vi "Control_cmd.vi"(6 "Arty-7 Error In":errorcluster, 7 "Control Command":u8 format="%b", 8 "Arty-7 VISA In":refnum<visa-resource-name>) -> (0 "Arty-7 Error out":errorcluster, 2 "WrReg Status":string, 3 "WrReg Done":bool, 5 "Arty-7 VISA out":refnum<visa-resource-name>)   [LabVIEW 2019]
uses:
  <vilib>/Utility/error.llb/DialogType.ctl
  Board_Global_Var.vi
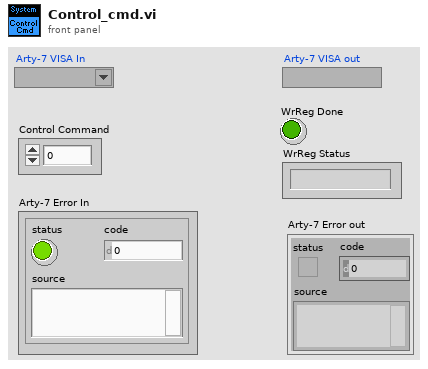
[diagram p1: front panel]
types:
  T1 = typedef "DialogType.ctl" = u16
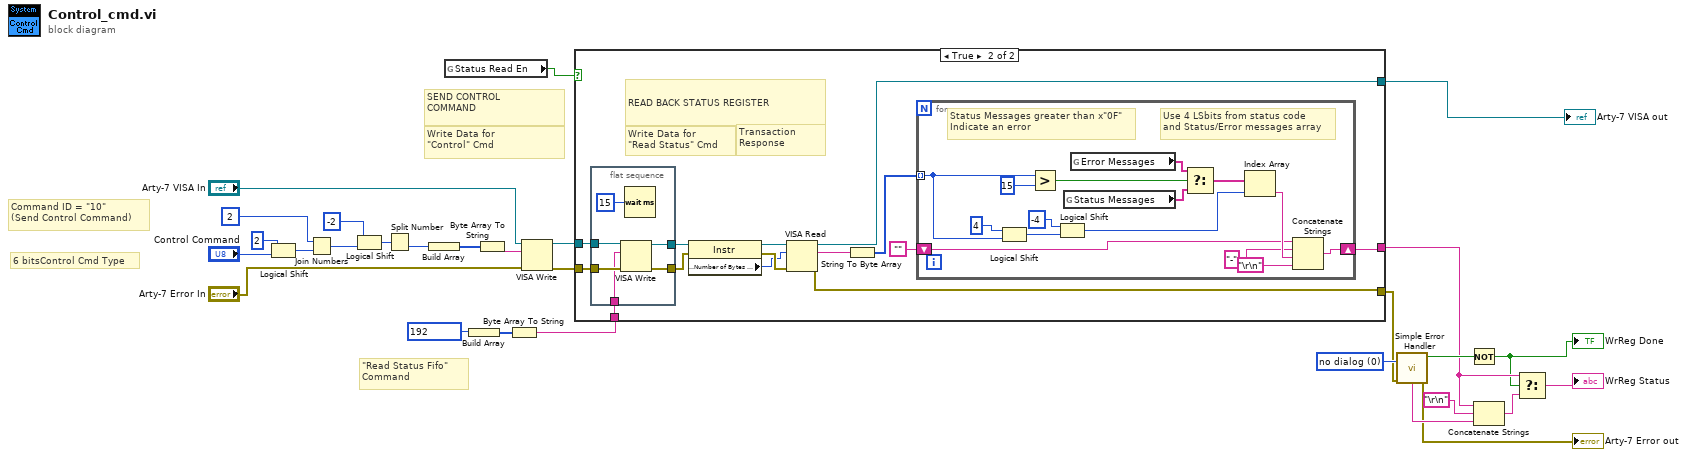
[diagram p0: block diagram]
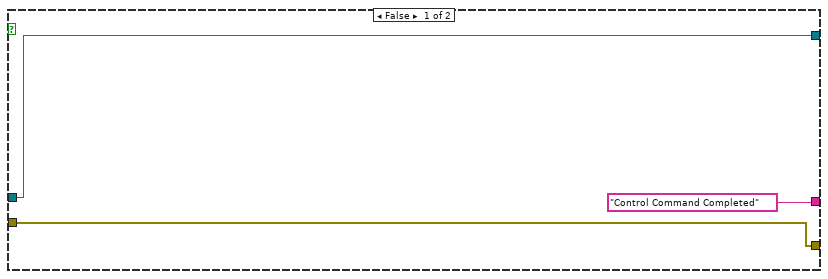
[diagram p2: hidden frame]
diagram:
  w14 = T1 0 items=["no dialog", "OK message", "continue or stop message", "OK message + warnings", "continue/stop + warnings"] ("type of dialog (OK msg:1)")
  # "\"Read Status Fifo\" \nCommand"
  # "SEND CONTROL\nCOMMAND"
  # "Write Data for \n\"Control\" Cmd"
  # "6 bitsControl Cmd Type"
  # "Command ID = \"10\" \n(Send Control Command)"
  n1 = Logical Shift(y=i16 2, x="Control Command") -> (x << y=w23:u8)
  n2 = Join Numbers(hi=u8 2, lo=w23) -> ((hi.lo)=w22:u16)
  n3 = Logical Shift(y=i16 -2, x=w22) -> (x << y=w26:u16)
  n4 = Split Number(x=w26) -> (lo(x)=w27:u8)  [unwired: 1 out]
  n5 = Build Array(w27) -> (w29:u8[])
  n6 = global read "Board_Global_Var.vi" "Status Read En"() -> (w1:bool)
  n7 = Build Array(u8 192) -> (w17:u8[])
  n8 = Byte Array To String(unsigned byte array=w29) -> (string=w28:string)
  n9 = Byte Array To String(unsigned byte array=w17) -> (string=w5:string)
  n10 = VISA Write(VISA resource name="Arty-7 VISA In", write buffer=w28, error in (no error)="Arty-7 Error In") -> (VISA resource name out=w7:refnum<visa-resource-name>, error out=w6:errorcluster)  [unwired: 1 out]
  n11 = case shown="True" w1 {
    tunnel: [w31 w46] -> w8
    tunnel: [w30 w45] -> w13
    tunnel: ["Control Command Completed" w43] -> w12
    tunnel: w7 -> [w31 w35]
    tunnel: w6 -> [w30 w34]
    tunnel: w5 -> [_ w33]
    frame False {
    }
    frame True {
      # "READ BACK STATUS REGISTER"
      # "Write Data for \n\"Read Status\" Cmd"
      # "Transaction \nResponse"
      n12 = flat-sequence {
        tunnel: [w52] -> w42
        tunnel: [w51] -> w41
        tunnel: w35 -> [w49]
        tunnel: w34 -> [w48]
        tunnel: w33 -> [w47]
        frame #0 {
          n13 = VISA Write(VISA resource name=w49, write buffer=w47, error in (no error)=w48) -> (VISA resource name out=w52:refnum<visa-resource-name>, error out=w51:errorcluster)  [unwired: 1 out]
          n14 = Wait (ms)(milliseconds to wait=u32 15) -> ()  [unwired: 1 out]
        }
      }
      n15 = property class="Instr"(reference=w42, error in=w41) -> (reference out=w40:refnum<visa-resource-name>, error out=w39:errorcluster, "Serial Settings:Number of Bytes at Serial Port"=w38:u32)
      n16 = VISA Read(VISA resource name=w40, byte count=w38, error in (no error)=w39) -> (VISA resource name out=w46:refnum<visa-resource-name>, read buffer=w44:string, error out=w45:errorcluster)  [unwired: 1 out]
      n17 = String To Byte Array(string=w44) -> (unsigned byte array=w37:u8[])
      n18 = for {
        tunnel: w37 -> [w57] mode=indexing
        shift-right: [w56] -> w43
        shift-left: "" -> [w55]
        # "Use 4 LSbits from status code \nand Status/Error messages array"
        # "Status Messages greater than x\"0F\"\nIndicate an error"
        n19 = Logical Shift(y=i16 4, x=w57) -> (x << y=w60:u8)
        n20 = Greater?(x=w57, y=u8 15) -> (0:w63:bool)
        n21 = Logical Shift(y=i16 -4, x=w60) -> (x << y=w61:u8)
        n22 = global read "Board_Global_Var.vi" "Status Messages"() -> (w64:string[])
        n23 = global read "Board_Global_Var.vi" "Error Messages"() -> (w65:string[])
        n24 = Select(t=w65, s=w63, f=w64) -> (s? t:f=w66:string[])
        n25 = Index Array(array=w66, index=w61) -> (element=w58:string)
        n26 = Concatenate Strings(w55, "-" ("string"), w58, "\r\n") -> (w56:string)
      }
    }
  }
  "Arty-7 VISA out" <- w8
  n27 = call <vilib>:"Simple Error Handler.vi"("type of dialog (OK msg:1)"=w14, "error in (no error)"=w13) -> ("error?"=w15:bool, "error out"=→"Arty-7 Error out":errorcluster, "message"=w10:string)  [unwired: 3 in, 2 out]
  n28 = Not(x=w15) -> (.not. x?=w3:bool)
  "WrReg Done" <- w3
  n29 = Concatenate Strings(w12, "\r\n", w10) -> (w9:string)
  n30 = Select(t=w12, s=w3, f=w9) -> (s? t:f=→"WrReg Status":string)
